vi "Register Dynamic Status Change Event.vi"() -> ()   [LabVIEW 2017]
doc: "------------- lvcsm -------------\n[CSMStates]\nItem 0 = \"Event Structure\"\nItem 1 = \"Idle\"\nItem 2 = \"CSM Documentation\"\nItem 3 = \"VI Reference\"\nItem 4 = \"Error Handler\"\nItem 5 = \"Critical Error\"\nItem 6 = \"Target Timeout Error\"\nItem 7 = \"Target Error\"\nItem 8 = \"Async Response\"\nItem 9 = \"Response\"\nItem 10 = \"Async Message Posted\"\nItem 11 = \"Initialize Core Data\"\nItem 12 = \"Exit\"\nItem 13 = \"Data: Initialize\"\nItem 14 = \"Data: Cleanup\"\nItem 15 = \"Events: Register\"\nItem 16 = \"Events: Unregister\"\nItem 17 = \"UI: Initialize\"\nItem 18 = \"UI: Cursor Set\"\nItem 19 = \"UI: Front Panel State\"\nItem 20 = \"Macro: Initialize\"\nItem 21 = \"Macro: Exit\"\nItem 22 = \"API: API1\"\nItem 23 = \"API: API2\"\nItem 24 = \"DoSth: DoA\"\nItem 25 = \"Update Status Changed\"\nItem 26 = \"DoSth: DoB\"\nItem 27 = \"Handler: Error Occurred\"\n\n[CSMStatus]"
uses:
  user.lib/_NEVSTOP/Communicable State Machine(CSM)/_Support/Common/Format Timestamp.vi
  user.lib/_NEVSTOP/Communicable State Machine(CSM)/_Polymophic/Build Synchronous Message with Arguments.vi
  user.lib/_NEVSTOP/Communicable State Machine(CSM)/Communicable State Machine.lvlib
  examples/NEVSTOP/Communicable State Machine(CSM)/1. Create a reuse Module/1. Create a reuse Module.lvlib
panel:
  in  "unRegister":bool
  in  "Register":bool
  out "State History 2":string
  in  "Start SubModule":bool
  out "State History":string
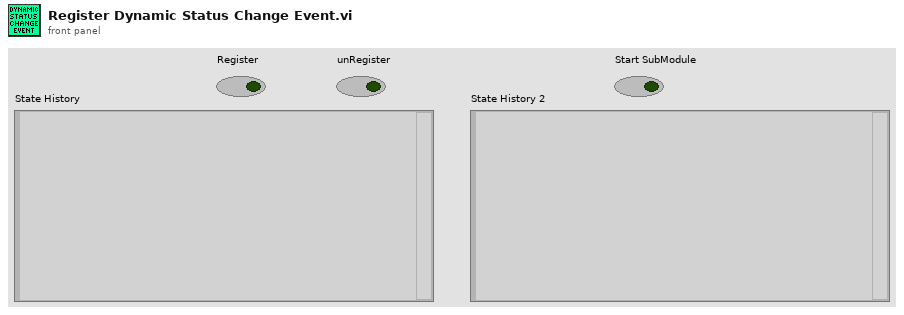
[diagram p1: front panel]
types:
  T1 = enum32{"Invalid", "Standard", "Closed", "Hidden", "Minimized", "Maximized"}
  T2 = enum32{"invalid app kind", "Development System", "Run Time System", "Student Edition", "Embedded LabVIEW", "Evaluation", "Custom"}
  T3 = typedef "Communicable State Machine.lvlib/_CSM_Response Source Message.ctl" = cluster{"‘State":string, "’Arguments":string, "’Error":errorcluster}
  T4 = cluster{"Current VI Reference":refnum<vi>, "Close Panel on Exit?":bool}
  T5 = cluster{"Core":cluster{"Current VI Reference":refnum<vi>, "Close Panel on Exit?":bool}, "Your Boolean data":bool, "Your string data":string}
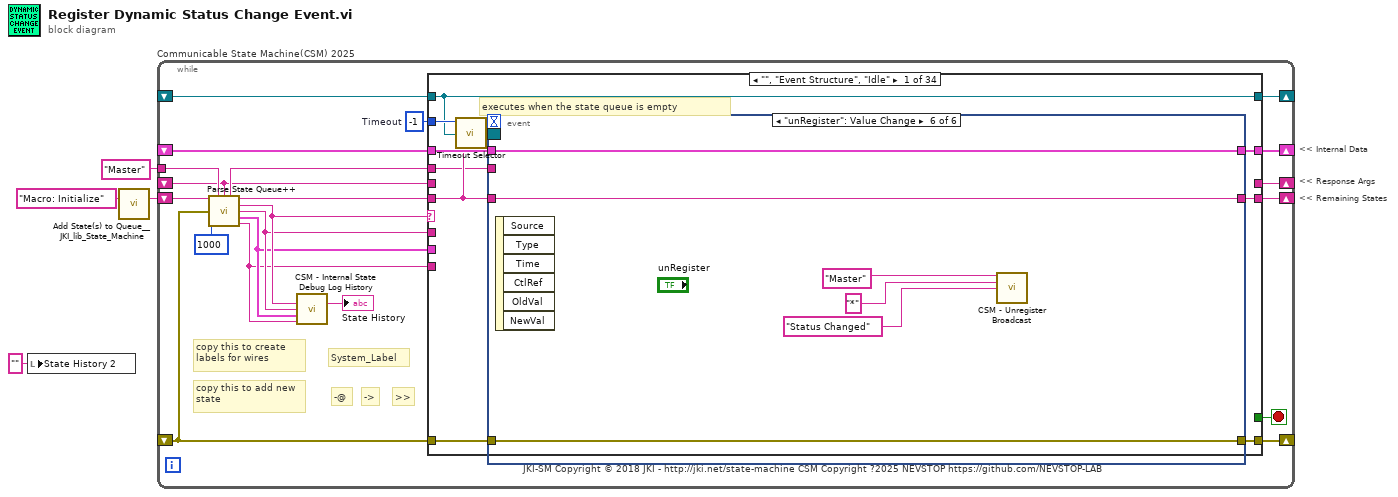
[diagram p0: block diagram]
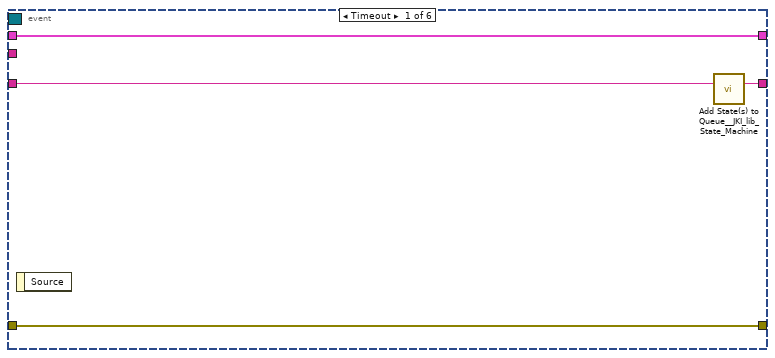
[diagram p2: hidden frame]
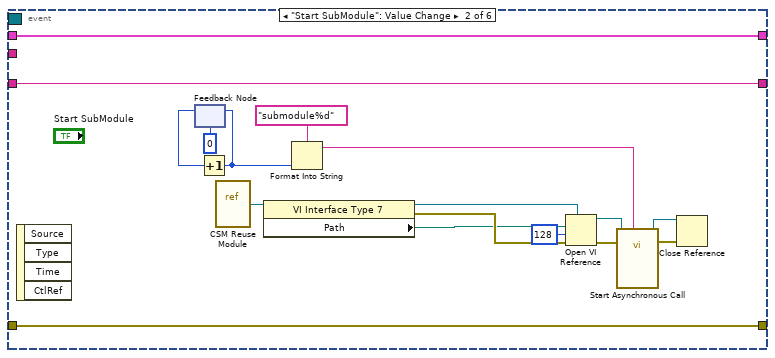
[diagram p3: hidden frame]
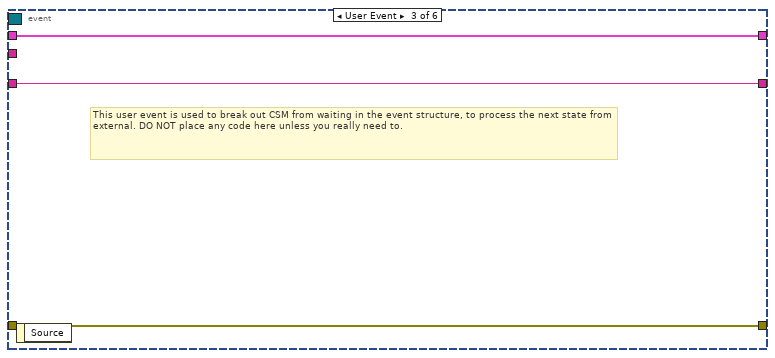
[diagram p4: hidden frame]
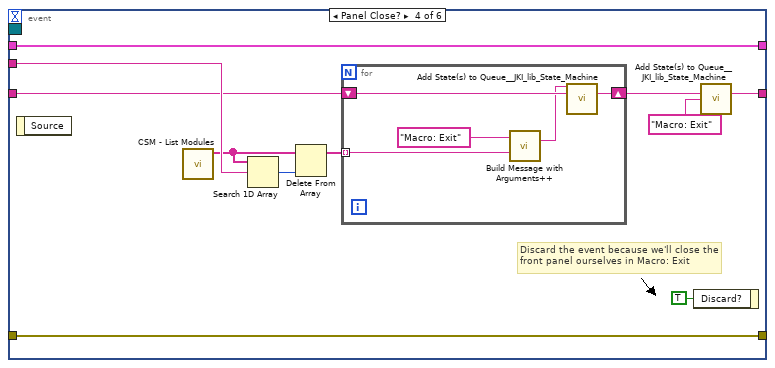
[diagram p5: hidden frame]
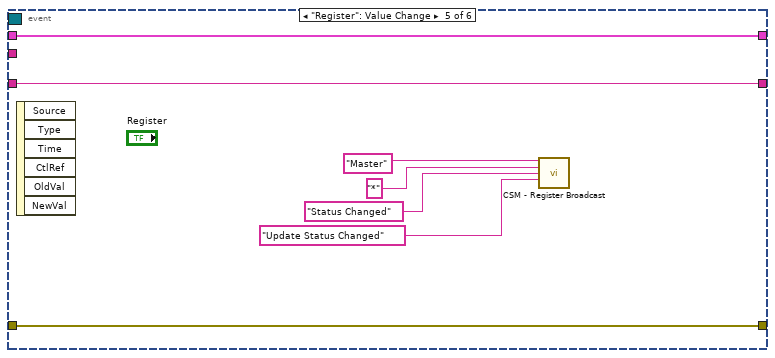
[diagram p6: hidden frame]
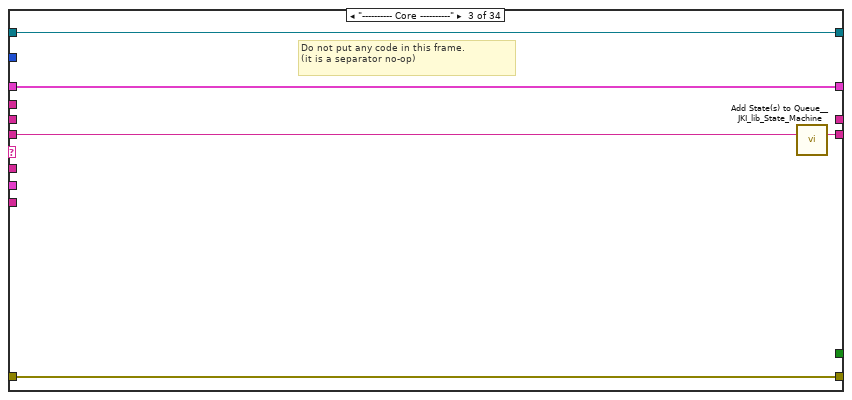
[diagram p8: hidden frame]
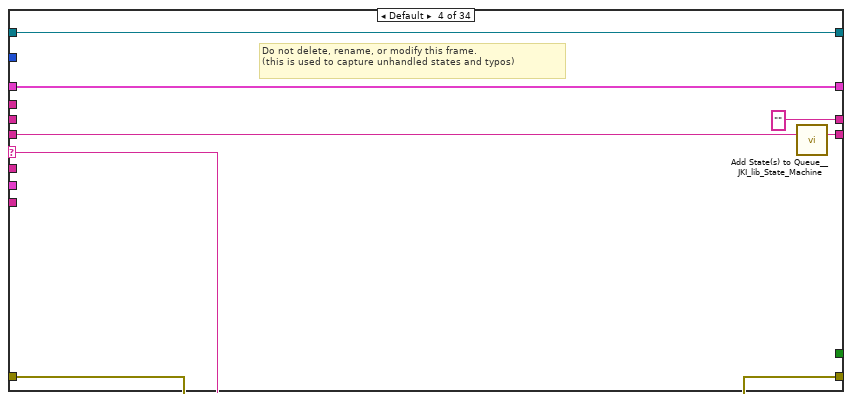
[diagram p9: hidden frame]
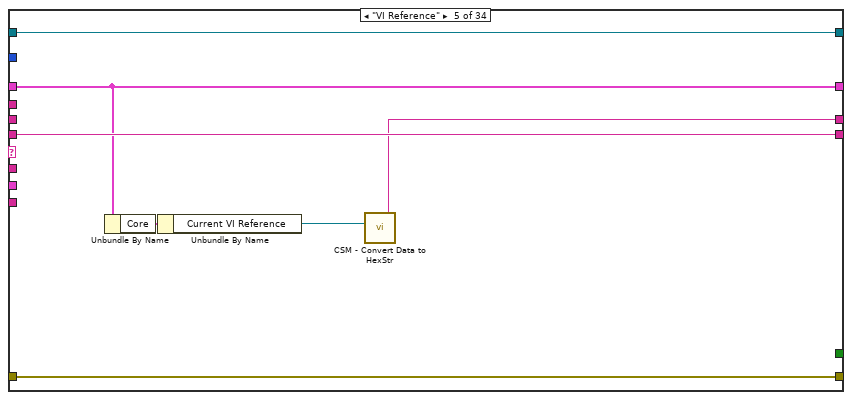
[diagram p10: hidden frame]
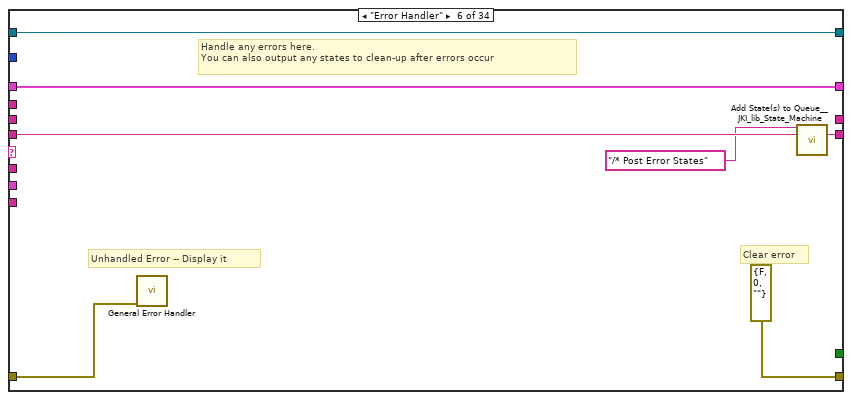
[diagram p11: hidden frame]
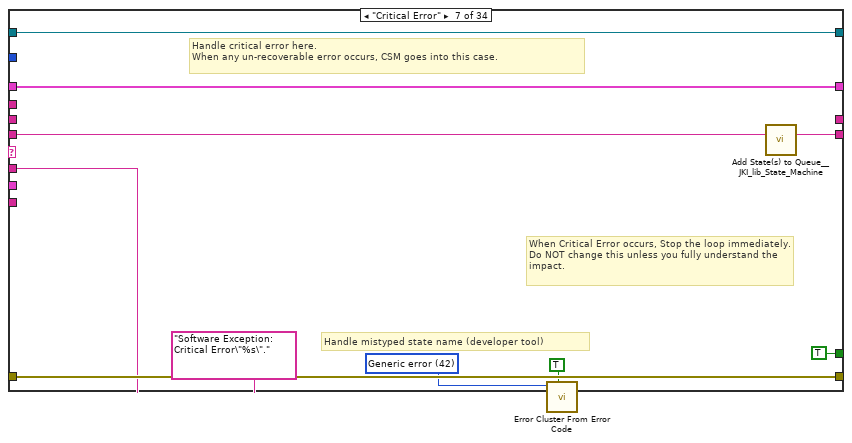
[diagram p12: hidden frame]
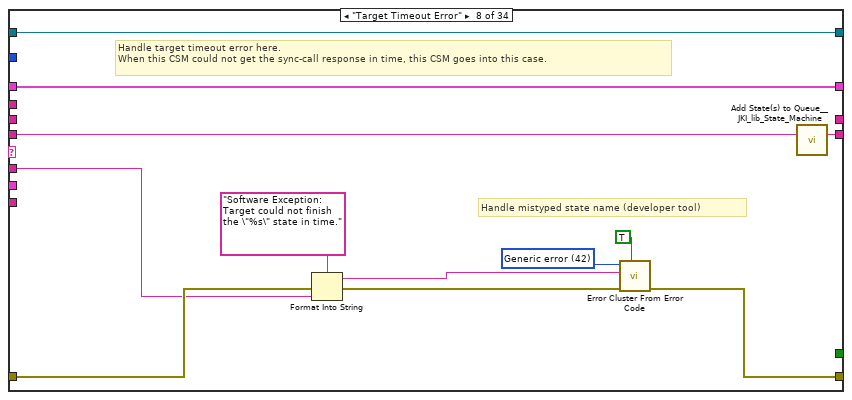
[diagram p13: hidden frame]
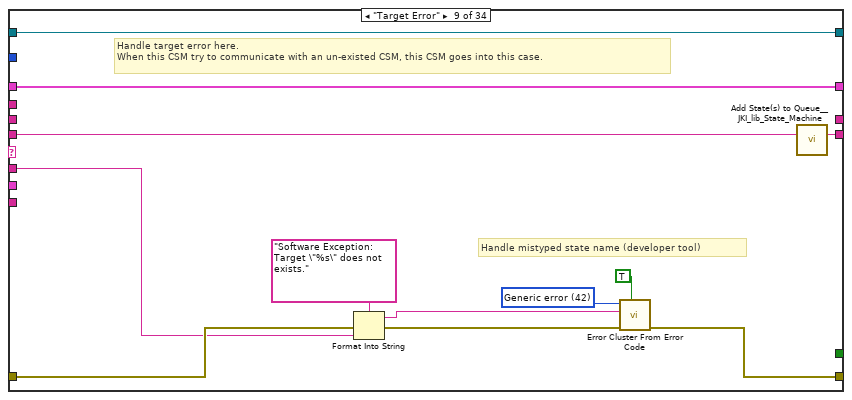
[diagram p14: hidden frame]
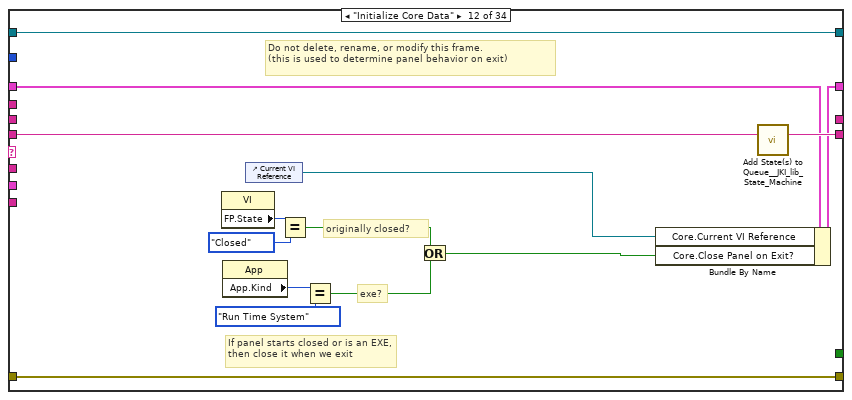
[diagram p17: hidden frame]
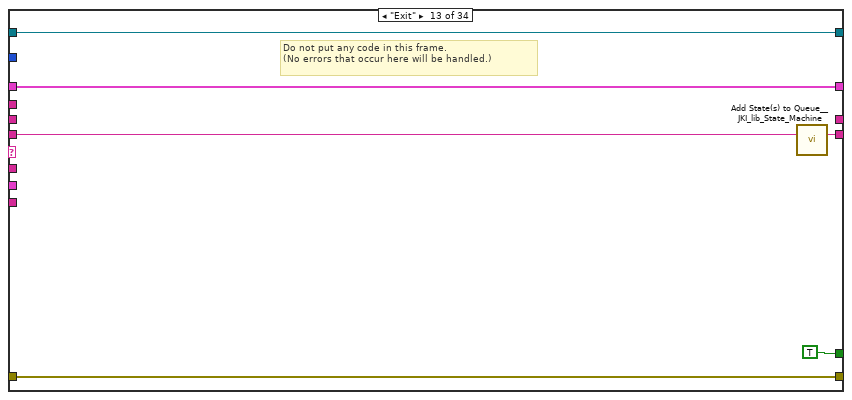
[diagram p18: hidden frame]
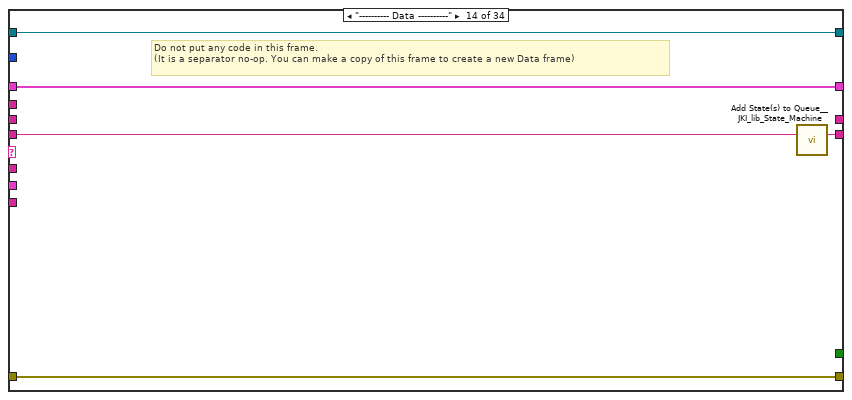
[diagram p19: hidden frame]
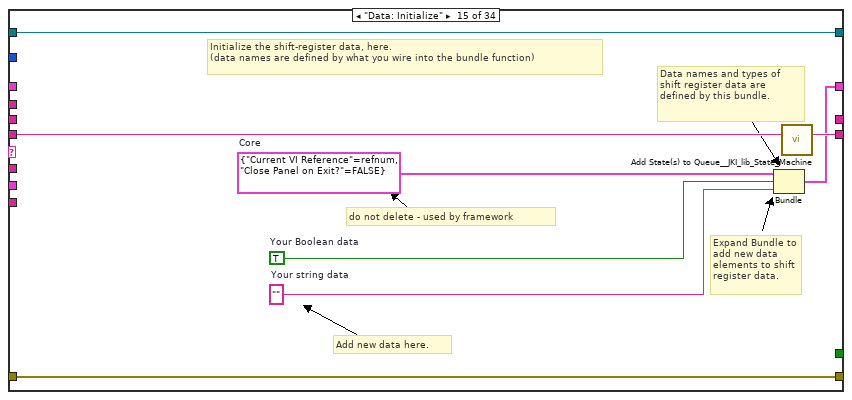
[diagram p20: hidden frame]
diagram:
  # "<< Internal Data"
  # "<< Response Args"
  # "<< Remaining States"
  n1 = local write "State History 2"("" ("State History 2")) -> ()
  n2 = call <vilib>:"Add State(s) to Queue__JKI_lib_State_Machine.vi"("State(s) in (\"\")"="Macro: Initialize") -> ("States Out"=w4:string)  [unwired: 14 in]
  n3 = while "Communicable State Machine(CSM) 2025" {
    shift-right: [w20] -> _
    shift-left: _ -> [w19]
    shift-right: [w23] -> _
    shift-left: _ -> [w17]
    shift-right: [w22] -> _
    shift-left: w4 -> [w24]
    tunnel: "Master" ("Name(\"\" to use uuid)") -> [w12]
    shift-right: [w15] -> _
    shift-left: _ -> [w6]
    shift-right: [w14] -> _
    shift-left: _ -> [w13]
    stop <- w21 stop-if-true
    w18 = -1  # Timeout
    # "JKI-SM Copyright © 2018 JKI - http://jki.net/state-machine CSM Copyright ?2025 NEVSTOP https://github.com/NEVSTOP-LAB"
    # "copy this to add new state"
    # ">>"
    # "->"
    # "-@"
    # "copy this to create labels for wires"
    # "System_Label"
    n4 = call "Parse State Queue++.vi"("State Queue"=w24, "Name (\"\" to Use UUID)"=w12, "Response Arguments"=w6, "Previous Error"=w17, "Response Timeout (-2 Use Global Settings)"=1000 ("Response Timeout(1000ms)")) -> ("Name Used"=w7:string, "Remaining States"=w25:string, "Current State"=w11:string, "Arguments"=w10:string, "Additional Information"=w9:T3, "Source CSM"=w8:string)  [unwired: 5 in]
    n5 = call "CSM - Internal State Debug Log History.vi"("State"=w11, "Arguments (\"\")"=w10, ">> Response Source Message >>"=w9, "Source (\"\")"=w8) -> ("Debug Log"=→"State History":string)  [unwired: 11 in]
    n6 = case shown="\"\", \"Event Structure\", \"Idle\"" w11 {
      selector: w11 -> [_ _ _ w100 _ _ _ _ _ _ _ _ _ _ _ _ _ _ _ _ _ _ _ _ _ _ _ _ _ _ _ _ _ _]
      tunnel: w25 -> [w27 w91 w97 w104 w116 w124 w134 w142 w154 w163 w167 w182 w188 w193 w201 w208 w213 w219 w223 w229 w234 w241 w253 w323 w329 w340 w343 w348 w354 w362 w368 w376 w383 w398]
      tunnel: w10 -> [_ _ _ _ _ _ w127 w138 w150 _ _ _ _ _ _ _ _ _ _ _ _ w236 w247 _ _ _ _ _ w351 _ _ w370 _ w395]
      tunnel: w19 -> [w34 w90 w94 w102 w115 w121 w135 w140 w152 w162 w166 w175 w186 w190 _ w203 w210 w218 w222 w226 w232 w239 w249 w320 w326 w337 w342 w347 w353 w359 w365 w375 w380 w397]
      tunnel: [w33 w92 w95 w106 w117 errorcluster {"status"=FALSE, "code"=0, "source"=""} ("error out") w136 w144 w156 w164 w168 w179 w185 w191 w198 w204 w211 w214 w221 w227 w231 w237 w250 w321 w327 w338 w344 w349 w355 w360 w366 w377 w381 w399] -> w23
      tunnel: w17 -> [w32 w92 w95 w105 w117 w120 w136 w143 w155 w164 w168 w179 w185 w191 w198 w205 w211 _ w224 w227 w231 w238 w251 w321 w327 w338 w344 w349 w355 w360 w366 w377 w381 w399]
      tunnel: [w35 w91 w96 w103 w116 w123 w133 w141 w153 w163 w167 w181 w187 w192 w200 w207 w212 w219 w223 w228 w233 w240 w252 w322 w328 w339 w343 w348 w354 w361 w367 w376 w382 w398] -> w22
      tunnel: [_ _ _ _ _ _ TRUE _ _ _ _ _ TRUE _ _ _ _ _ _ _ _ _ _ _ _ _ _ _ _ _ _ _ _ _] -> w21
      tunnel: [w31 w90 w94 w102 w115 w121 w135 w140 w152 w162 w166 w180 w186 w190 w199 w203 w210 w218 w222 w226 w232 w239 w249 w320 w326 w337 w342 w347 w353 w359 w365 w375 w380 w397] -> w20
      tunnel: w18 -> [w30 _ _ _ _ _ _ _ _ _ _ _ _ _ _ _ _ _ _ _ _ _ _ _ _ _ _ _ _ _ _ _ _ _]
      tunnel: w8 -> [_ _ _ _ _ _ _ _ _ _ _ _ _ _ _ _ _ _ _ _ _ _ _ _ _ _ _ _ _ _ _ w371 _ w390]
      tunnel: w9 -> [_ _ _ _ _ _ _ _ _ _ _ _ _ _ _ _ _ _ _ _ _ _ _ _ _ _ _ _ _ _ _ _ _ w389]
      tunnel: [_ _ _ "" w111 _ _ _ _ _ _ _ _ _ _ _ _ _ _ _ _ _ _ _ _ _ _ "API1 Response" w350 _ "DoA Finished" _ "DoB Finished" _] -> w15
      tunnel: [w29 w89 w93 w98 w114 w118 w125 w137 w149 w161 w165 w169 w183 w189 w194 w202 w209 w217 w220 w225 w230 w235 w246 w319 w324 w330 w341 w346 w352 w358 w364 w374 w379 w396] -> w14
      tunnel: w13 -> [w29 w89 w93 w98 w114 w118 w125 w137 w149 w161 w165 w169 w183 w189 w194 w202 w209 _ w220 w225 w230 w235 w246 w319 w324 w330 w341 w346 w352 w358 w364 w374 w379 w396]
      tunnel: w7 -> [w26 _ _ _ _ _ _ _ _ _ _ _ _ _ _ _ _ w216 _ _ _ _ _ _ _ _ _ _ _ _ _ _ _ _]
      tunnel: w6 -> [_ _ _ _ _ _ _ _ _ _ _ _ _ _ _ _ _ _ _ _ _ _ _ _ _ _ _ _ _ _ _ _ _ _]
      frame "", "Event Structure", "Idle" {
        # "executes when the state queue is empty"
        n7 = call "Timeout Selector.vi"("Remaining States"=w27, "Timeout Expected"=w30) -> ("Timeout"=w28:i32)  [unwired: 5 in]
        n8 = event shown="[5] \"unRegister\": Value Change" {
          selector: w29 -> [_ _ _ _ _ _]
          dyn-events: _ -> [_ _ _ _ _ _]
          timeout: w28 -> [_ _ _ _ _ _]
          tunnel: w27 -> [w39 w56 w58 w61 w82 w88]
          tunnel: [w38 w56 w58 w70 w82 w88] -> w35
          tunnel: w34 -> [w36 w54 w59 w68 w80 w86]
          tunnel: [w37 w55 w57 w69 w81 w87] -> w33
          tunnel: w32 -> [w37 w55 w57 w69 w81 w87]
          tunnel: [w36 w54 w59 w68 w80 w86] -> w31
          tunnel: w26 -> [_ _ _ w66 _ _]
          event Timeout {
            n9 = event-data() -> ()  [unwired: 1 in, 1 out]
            n10 = call <vilib>:"Add State(s) to Queue__JKI_lib_State_Machine.vi"("State(s) in (\"\")"=w39) -> ("States Out"=w38:string)  [unwired: 14 in]
          }
          event "Start SubModule": Value Change {
            n11 = event-data() -> ()  [unwired: 1 in, 4 out]
            n12 = feedback #1(0 ("Response Timeout(1000ms)")) -> (w52:i32)
            n13 = Increment(x=w52) -> (x+1=w42:i32)
            n14 = feedback-in #1(w42) -> ()
            n15 = vi-ref "CSM Reuse Module.vi"() -> (w44:refnum<vi>)
            n16 = property class="VI Interface Type 7"(reference=w44) -> (reference out=w48:refnum<vi>, error out=w46:errorcluster, "Path"=w45:path)  [unwired: 1 in]
            n17 = Format Into String(format string="submodule%d", w42) -> (resulting string=w40:string)  [unwired: 2 in, 1 out]
            n18 = Open VI Reference(type specifier VI Refnum (for type only)=w48, vi path=w45, options=128, error in (no error)=w46) -> (vi reference=w47:refnum<vi>, error out=w43:errorcluster)  [unwired: 2 in]
            n19 = call-by-ref "Start Asynchronous Call"(reference=w47, error in=w43, "Name(\"\" to use uuid)"=w40) -> (reference out=w50:refnum<vi>, error out=w49:errorcluster)  [unwired: 11 in]
            n20 = Close Reference(reference=w50, error in (no error)=w49) -> ()  [unwired: 1 out]
          }
          event User Event {
            # "This user event is used to break out CSM from waiting in the event structure, to process the next state from external. DO NOT place any code here unless you really need to."
            n21 = event-data() -> ()  [unwired: 1 in, 1 out]
          }
          event Panel Close? {
            # "Discard the event because we'll close the front panel ourselves in Macro: Exit"
            n22 = event-data() -> ()  [unwired: 1 in, 1 out]
            n23 = call "CSM - List Modules.vi"() -> ("Module Names"=w65:string[])  [unwired: 10 in, 1 out]
            n24 = Search 1D Array(1D array=w65, element=w66) -> (index of element=w64:i32)  [unwired: 1 in]
            n25 = Delete From Array(array=w65, index=w64) -> (array with subset deleted=w63:string[])  [unwired: 1 in, 1 out]
            n26 = for {
              tunnel: w63 -> [w75] mode=indexing
              shift-right: [w73] -> w62
              shift-left: w61 -> [w72]
              n27 = call-poly "Build Message with Arguments++.vi"("State With Arguments"="Macro: Exit", "Target Module (\"\")"=w75) -> ("CSM Message String"=w71:string)  [unwired: 13 in]
              n28 = call <vilib>:"Add State(s) to Queue__JKI_lib_State_Machine.vi"("State(s) in Front (\"\")"=w71, "State(s) in (\"\")"=w72) -> ("States Out"=w73:string)  [unwired: 13 in]
            }
            n29 = event-data("Discard?"=TRUE) -> ()  [unwired: 1 in, 1 out]
            n30 = call <vilib>:"Add State(s) to Queue__JKI_lib_State_Machine.vi"("State(s) in (\"\")"=w62, "State(s) at Back (\"\")"="Macro: Exit") -> ("States Out"=w70:string)  [unwired: 13 in]
          }
          event "Register": Value Change {
            n31 = event-data() -> ()  [unwired: 1 in, 6 out]
            n32 = call "CSM - Register Broadcast.vi"("CSM Name(Empty for Broadcast Event)"="Master" ("Source CSM Name"), "Source CSM Name (* as Default)"="*" ("Name(\"\" to use uuid)"), "Trigger"="Status Changed" ("Message"), "API (If \"\", Same as Trigger)"="Update Status Changed" ("Response Message (if \"\", same as Source Message)")) -> ()  [unwired: 10 in, 2 out]
          }
          event "unRegister": Value Change {
            n33 = event-data() -> ()  [unwired: 1 in, 6 out]
            n34 = call "CSM - Unregister Broadcast.vi"("CSM Name(Empty for Broadcast Event)"="Master" ("Source CSM Name"), "Source CSM Name (* as Default)"="*" ("Name(\"\" to use uuid)"), "Trigger"="Status Changed" ("Message")) -> ()  [unwired: 11 in, 2 out]
          }
        }
      }
      frame "CSM Documentation" {
        # "CSM Documentation"
      }
      frame "---------- Core ----------" {
        # "Do not put any code in this frame.\n(it is a separator no-op)"
        n35 = call <vilib>:"Add State(s) to Queue__JKI_lib_State_Machine.vi"("State(s) in (\"\")"=w97) -> ("States Out"=w96:string)  [unwired: 14 in]
      }
      frame Default {
        w109 = 42 items=["No error", "Argument error", "Memory is full", "Out of zone", "End of file", "File already open", "Generic file I/O error", "File not found", "File permission error", "Disk is full", "Duplicate path", "Too many files open", "System feature not enabled", "Resource file not found", "Cannot add resource", "Resource not found", "Image not found", "Image memory error", "Pen does not exist", "Config type invalid", "Config token not found", "Config parse error", "Config memory error", "Bad external code format", "Bad external code offset", "External code not present", "Null window", "Destroy window error", "Null menu", "Print aborted", "Bad print record", "Print driver error", "Windows error during printing", "Memory error during printing", "Print dialog error", "Generic print error", "Invalid device refnum", "Device not found", "Device parameter error", "Device unit error", "Cannot open device", "Device call aborted", "Generic error", "Cancelled by user", "Object ID too low", "Object ID too high", "Object not in heap", "Unknown heap", "Unknown object (invalid DefProc)", "Unknown object (DefProc not in table)", "Message out of range", "Invalid (null) method", "Unknown message", "Manager call not supported", "Bad address", "Network operation in progress", "Network operation timed out", "Connection is busy", "Network attribute not supported", "Network error", "Address in use", "System out of memory", "Connection aborted", "Connection refused", "Not connected", "Already connected", "Connection closed", "Initialization error (interapplication manager)", "Bad occurrence", "Wait on unbound occurrence handler", "Occurrence queue overflow", "Datalog type conflict", "Unused", "Unrecognized type (interapplication manager)", "Memory corrupt", "Failed to make temporary DLL", "Old CIN version", "Drag socket not found", "Failed to load drop-object", "Failed to register OLE object", "Failed to release OLE object", "Format specifier type mismatch", "Unknown format specifier", "Too few format specifiers", "Too many format specifiers", "Scan failed", "Newer CIN version", "Error converting to variant", "Runtime menu error", "Password tampered", "Variant attribute not found", "Incompatible variant data type", "Event data is not available", "Event Store is not present", "Occurrence is not found", "Event Queue is not created", "Event info is not available", "Refnum passed is NULL", "Error retrieving Class GUID", "Error retrieving CoClass GUID", "Error retrieving TypeLib GUID.", "Bad built application magic bytes.", "Specific driver is different from the specific driver associated with the Logical Name.", "There is no session opened to the class driver.", "Max Error", "MAX - Error with config objects", "MAX - Error loading configuration", "MAX - Group not supported"]
        # "Do not delete, rename, or modify this frame.\n(this is used to capture unhandled states and typos)"
        # "Handle mistyped state name (developer tool)"
        n36 = Format Into String(format string="Software Exception: Unhandled State \"%s\"." ("message"), error in=w105, w100) -> (resulting string=w108:string, error out=w107:errorcluster)  [unwired: 1 in]
        n37 = call <vilib>:"Error Cluster From Error Code.vi"("show call chain? (False)"=TRUE, "error in (no error)"=w107, "error message (\"\")"=w108, "error code (0)"=w109) -> ("error out"=w106:errorcluster)  [unwired: 5 in]
        n38 = call <vilib>:"Add State(s) to Queue__JKI_lib_State_Machine.vi"("State(s) in (\"\")"=w104) -> ("States Out"=w103:string)  [unwired: 14 in]
      }
      frame "VI Reference" {
        n39 = Unbundle By Name(w115) -> ("Core"=w113:T4)
        n40 = Unbundle By Name(w113) -> ("Current VI Reference"=w112:refnum<vi>)
        n41 = call "CSM - Convert Data to HexStr.vi"("Variant"=w112) -> ("HEX String (0-9,A-F)"=w111:string)  [unwired: 8 in]
      }
      frame "Error Handler" {
        # "Unhandled Error -- Display it"
        # "Handle any errors here.\nYou can also output any states to clean-up after errors occur"
        # "Clear error"
        n42 = call <vilib>:"General Error Handler.vi"("error in (no error)"=w120) -> ()  [unwired: 10 in, 5 out]
        n43 = call <vilib>:"Add State(s) to Queue__JKI_lib_State_Machine.vi"("State(s) in Front (\"\")"="/* Post Error States", "State(s) in (\"\")"=w124) -> ("States Out"=w123:string)  [unwired: 13 in]
      }
      frame "Critical Error" {
        w131 = 42 items=["No error", "Argument error", "Memory is full", "Out of zone", "End of file", "File already open", "Generic file I/O error", "File not found", "File permission error", "Disk is full", "Duplicate path", "Too many files open", "System feature not enabled", "Resource file not found", "Cannot add resource", "Resource not found", "Image not found", "Image memory error", "Pen does not exist", "Config type invalid", "Config token not found", "Config parse error", "Config memory error", "Bad external code format", "Bad external code offset", "External code not present", "Null window", "Destroy window error", "Null menu", "Print aborted", "Bad print record", "Print driver error", "Windows error during printing", "Memory error during printing", "Print dialog error", "Generic print error", "Invalid device refnum", "Device not found", "Device parameter error", "Device unit error", "Cannot open device", "Device call aborted", "Generic error", "Cancelled by user", "Object ID too low", "Object ID too high", "Object not in heap", "Unknown heap", "Unknown object (invalid DefProc)", "Unknown object (DefProc not in table)", "Message out of range", "Invalid (null) method", "Unknown message", "Manager call not supported", "Bad address", "Network operation in progress", "Network operation timed out", "Connection is busy", "Network attribute not supported", "Network error", "Address in use", "System out of memory", "Connection aborted", "Connection refused", "Not connected", "Already connected", "Connection closed", "Initialization error (interapplication manager)", "Bad occurrence", "Wait on unbound occurrence handler", "Occurrence queue overflow", "Datalog type conflict", "Unused", "Unrecognized type (interapplication manager)", "Memory corrupt", "Failed to make temporary DLL", "Old CIN version", "Drag socket not found", "Failed to load drop-object", "Failed to register OLE object", "Failed to release OLE object", "Format specifier type mismatch", "Unknown format specifier", "Too few format specifiers", "Too many format specifiers", "Scan failed", "Newer CIN version", "Error converting to variant", "Runtime menu error", "Password tampered", "Variant attribute not found", "Incompatible variant data type", "Event data is not available", "Event Store is not present", "Occurrence is not found", "Event Queue is not created", "Event info is not available", "Refnum passed is NULL", "Error retrieving Class GUID", "Error retrieving CoClass GUID", "Error retrieving TypeLib GUID.", "Bad built application magic bytes.", "Specific driver is different from the specific driver associated with the Logical Name.", "There is no session opened to the class driver.", "Max Error", "MAX - Error with config objects", "MAX - Error loading configuration", "MAX - Group not supported"]
        # "Handle critical error here.\nWhen any un-recoverable error occurs, CSM goes into this case."
        # "When Critical Error occurs, Stop the loop immediately. Do NOT change this unless you fully understand the impact."
        # "Handle mistyped state name (developer tool)"
        n44 = Format Into String(format string="Software Exception: Critical Error\"%s\"." ("message"), w127) -> (resulting string=w130:string, error out=w129:errorcluster)  [unwired: 2 in]
        n45 = call <vilib>:"Error Cluster From Error Code.vi"("show call chain? (False)"=TRUE, "error in (no error)"=w129, "error message (\"\")"=w130, "error code (0)"=w131) -> ()  [unwired: 5 in, 1 out]
        n46 = call <vilib>:"Add State(s) to Queue__JKI_lib_State_Machine.vi"("State(s) in (\"\")"=w134) -> ("States Out"=w133:string)  [unwired: 14 in]
      }
      frame "Target Timeout Error" {
        w147 = 42 items=["No error", "Argument error", "Memory is full", "Out of zone", "End of file", "File already open", "Generic file I/O error", "File not found", "File permission error", "Disk is full", "Duplicate path", "Too many files open", "System feature not enabled", "Resource file not found", "Cannot add resource", "Resource not found", "Image not found", "Image memory error", "Pen does not exist", "Config type invalid", "Config token not found", "Config parse error", "Config memory error", "Bad external code format", "Bad external code offset", "External code not present", "Null window", "Destroy window error", "Null menu", "Print aborted", "Bad print record", "Print driver error", "Windows error during printing", "Memory error during printing", "Print dialog error", "Generic print error", "Invalid device refnum", "Device not found", "Device parameter error", "Device unit error", "Cannot open device", "Device call aborted", "Generic error", "Cancelled by user", "Object ID too low", "Object ID too high", "Object not in heap", "Unknown heap", "Unknown object (invalid DefProc)", "Unknown object (DefProc not in table)", "Message out of range", "Invalid (null) method", "Unknown message", "Manager call not supported", "Bad address", "Network operation in progress", "Network operation timed out", "Connection is busy", "Network attribute not supported", "Network error", "Address in use", "System out of memory", "Connection aborted", "Connection refused", "Not connected", "Already connected", "Connection closed", "Initialization error (interapplication manager)", "Bad occurrence", "Wait on unbound occurrence handler", "Occurrence queue overflow", "Datalog type conflict", "Unused", "Unrecognized type (interapplication manager)", "Memory corrupt", "Failed to make temporary DLL", "Old CIN version", "Drag socket not found", "Failed to load drop-object", "Failed to register OLE object", "Failed to release OLE object", "Format specifier type mismatch", "Unknown format specifier", "Too few format specifiers", "Too many format specifiers", "Scan failed", "Newer CIN version", "Error converting to variant", "Runtime menu error", "Password tampered", "Variant attribute not found", "Incompatible variant data type", "Event data is not available", "Event Store is not present", "Occurrence is not found", "Event Queue is not created", "Event info is not available", "Refnum passed is NULL", "Error retrieving Class GUID", "Error retrieving CoClass GUID", "Error retrieving TypeLib GUID.", "Bad built application magic bytes.", "Specific driver is different from the specific driver associated with the Logical Name.", "There is no session opened to the class driver.", "Max Error", "MAX - Error with config objects", "MAX - Error loading configuration", "MAX - Group not supported"]
        # "Handle target timeout error here.\nWhen this CSM could not get the sync-call response in time, this CSM goes into this case."
        # "Handle mistyped state name (developer tool)"
        n47 = Format Into String(format string="Software Exception: Target could not finish the \"%s\" state in time." ("message"), error in=w143, w138) -> (resulting string=w146:string, error out=w145:errorcluster)  [unwired: 1 in]
        n48 = call <vilib>:"Error Cluster From Error Code.vi"("show call chain? (False)"=TRUE, "error in (no error)"=w145, "error message (\"\")"=w146, "error code (0)"=w147) -> ("error out"=w144:errorcluster)  [unwired: 5 in]
        n49 = call <vilib>:"Add State(s) to Queue__JKI_lib_State_Machine.vi"("State(s) in (\"\")"=w142) -> ("States Out"=w141:string)  [unwired: 14 in]
      }
      frame "Target Error" {
        w159 = 42 items=["No error", "Argument error", "Memory is full", "Out of zone", "End of file", "File already open", "Generic file I/O error", "File not found", "File permission error", "Disk is full", "Duplicate path", "Too many files open", "System feature not enabled", "Resource file not found", "Cannot add resource", "Resource not found", "Image not found", "Image memory error", "Pen does not exist", "Config type invalid", "Config token not found", "Config parse error", "Config memory error", "Bad external code format", "Bad external code offset", "External code not present", "Null window", "Destroy window error", "Null menu", "Print aborted", "Bad print record", "Print driver error", "Windows error during printing", "Memory error during printing", "Print dialog error", "Generic print error", "Invalid device refnum", "Device not found", "Device parameter error", "Device unit error", "Cannot open device", "Device call aborted", "Generic error", "Cancelled by user", "Object ID too low", "Object ID too high", "Object not in heap", "Unknown heap", "Unknown object (invalid DefProc)", "Unknown object (DefProc not in table)", "Message out of range", "Invalid (null) method", "Unknown message", "Manager call not supported", "Bad address", "Network operation in progress", "Network operation timed out", "Connection is busy", "Network attribute not supported", "Network error", "Address in use", "System out of memory", "Connection aborted", "Connection refused", "Not connected", "Already connected", "Connection closed", "Initialization error (interapplication manager)", "Bad occurrence", "Wait on unbound occurrence handler", "Occurrence queue overflow", "Datalog type conflict", "Unused", "Unrecognized type (interapplication manager)", "Memory corrupt", "Failed to make temporary DLL", "Old CIN version", "Drag socket not found", "Failed to load drop-object", "Failed to register OLE object", "Failed to release OLE object", "Format specifier type mismatch", "Unknown format specifier", "Too few format specifiers", "Too many format specifiers", "Scan failed", "Newer CIN version", "Error converting to variant", "Runtime menu error", "Password tampered", "Variant attribute not found", "Incompatible variant data type", "Event data is not available", "Event Store is not present", "Occurrence is not found", "Event Queue is not created", "Event info is not available", "Refnum passed is NULL", "Error retrieving Class GUID", "Error retrieving CoClass GUID", "Error retrieving TypeLib GUID.", "Bad built application magic bytes.", "Specific driver is different from the specific driver associated with the Logical Name.", "There is no session opened to the class driver.", "Max Error", "MAX - Error with config objects", "MAX - Error loading configuration", "MAX - Group not supported"]
        # "Handle target error here.\nWhen this CSM try to communicate with an un-existed CSM, this CSM goes into this case."
        # "Handle mistyped state name (developer tool)"
        n50 = Format Into String(format string="Software Exception: Target \"%s\" does not exists." ("message"), error in=w155, w150) -> (resulting string=w158:string, error out=w157:errorcluster)  [unwired: 1 in]
        n51 = call <vilib>:"Error Cluster From Error Code.vi"("show call chain? (False)"=TRUE, "error in (no error)"=w157, "error message (\"\")"=w158, "error code (0)"=w159) -> ("error out"=w156:errorcluster)  [unwired: 5 in]
        n52 = call <vilib>:"Add State(s) to Queue__JKI_lib_State_Machine.vi"("State(s) in (\"\")"=w154) -> ("States Out"=w153:string)  [unwired: 14 in]
      }
      frame "Async Response", "Response" {
        # "Handle Async-call Response (\"Async Response\" for ->)"
        # "Handle Sync-call Response (\"Response\" for @)"
        # "After Message is executed, CSM goes to this state for receive the response. \n    For Async Message(->), \"Async Response\" is used. This CSM will goes to \"Async Message Posted\" immediately and receive the \"Async Response\" after the callee finishes the message.\n    For Sync Message(@),  This CSM will wait until the message is done and immediately goes to \"Response\""
      }
      frame "Async Message Posted" {
        # "Handle post action for async message (->)."
        # "After Async Message is posted (->), CSM goes to this state for post-action. You can use Argument - State to tell which Async Message is called."
      }
      frame "Initialize Core Data" {
        # "Do not delete, rename, or modify this frame.\n(this is used to determine panel behavior on exit)"
        # "originally closed?"
        # "exe?"
        # "If panel starts closed or is an EXE, then close it when we exit"
        n53 = property class="VI"() -> ("FP.State"=w172:T1)  [unwired: 2 in, 2 out]
        n54 = property class="App"() -> ("App.Kind"=w178:T2)  [unwired: 2 in, 2 out]
        n55 = control-ref of="Current VI Reference"() -> (w173:refnum<vi>)
        n56 = Equal?(x=w172, y=T1."Closed" ("Front Panel Window:State")) -> (x = y?=w170:bool)
        n57 = Equal?(x=w178, y=T2."Run Time System" ("Application:Kind")) -> (x = y?=w176:bool)
        n58 = Or(x=w170, y=w176) -> (x .or. y?=w174:bool)
        n59 = Bundle By Name(cluster=w175, "Core.Current VI Reference"=w173, "Core.Close Panel on Exit?"=w174) -> (w180:T5)
        n60 = call <vilib>:"Add State(s) to Queue__JKI_lib_State_Machine.vi"("State(s) in (\"\")"=w182) -> ("States Out"=w181:string)  [unwired: 14 in]
      }
      frame "Exit" {
        # "Do not put any code in this frame.\n(No errors that occur here will be handled.)"
        n61 = call <vilib>:"Add State(s) to Queue__JKI_lib_State_Machine.vi"("State(s) in (\"\")"=w188) -> ("States Out"=w187:string)  [unwired: 14 in]
      }
      frame "---------- Data ----------" {
        # "Do not put any code in this frame.\n(It is a separator no-op. You can make a copy of this frame to create a new Data frame)"
        n62 = call <vilib>:"Add State(s) to Queue__JKI_lib_State_Machine.vi"("State(s) in (\"\")"=w193) -> ("States Out"=w192:string)  [unwired: 14 in]
      }
      frame "Data: Initialize" {
        w195 = T4 {"Current VI Reference"=refnum, "Close Panel on Exit?"=FALSE}  # Core
        w197 = TRUE  # Your Boolean data
        w196 = ""  # Your string data
        # "do not delete - used by framework"
        # "Expand Bundle to add new data elements to shift register data."
        # "Add new data here."
        # "Data names and types of shift register data are defined by this bundle."
        # "Initialize the shift-register data, here.\n(data names are defined by what you wire into the bundle function)"
        n63 = Bundle("Core"=w195, "Your Boolean data"=w197, "Your string data"=w196) -> (w199:T5)  [unwired: 1 in]
        n64 = call <vilib>:"Add State(s) to Queue__JKI_lib_State_Machine.vi"("State(s) in (\"\")"=w201) -> ("States Out"=w200:string)  [unwired: 14 in]
      }
      frame "Data: Cleanup" {
        # "Cleanup any data and references, here.\n(this is called automatically, by the Macro: Exit)"
        n65 = Unbundle By Name(w203) -> ("Core.Current VI Reference"=w206:refnum<vi>)
        n66 = Close Reference(reference=w206, error in (no error)=w205) -> (error out=w204:errorcluster)
        n67 = call <vilib>:"Add State(s) to Queue__JKI_lib_State_Machine.vi"("State(s) in (\"\")"=w208) -> ("States Out"=w207:string)  [unwired: 14 in]
      }
      frame "---------- Events ----------" {
        # "Do not put any code in this frame.\n(It is a separator no-op. You can make a copy of this frame to create a new UI frame)"
        n68 = call <vilib>:"Add State(s) to Queue__JKI_lib_State_Machine.vi"("State(s) in (\"\")"=w213) -> ("States Out"=w212:string)  [unwired: 14 in]
      }
      frame "Events: Register" {
        # "Register message event to break Waiting in Event structure."
        n69 = call "CSM - Get New State Notifier Event.vi"("Name (\"\" to Use UUID)"=w216) -> ("error out"=w214:errorcluster, "New State Notifier Event"=w215:refnum<user-event>)  [unwired: 9 in]
        n70 = register-events(w215) -> (reference out=w217:refnum<event-registration>)  [unwired: 2 in, 1 out]
      }
      frame "Events: Unregister" {
        n71 = Unregister For Events(event registration refnum=w220, error in=w224) -> (error out=w221:errorcluster)
      }
      frame "---------- UI ----------" {
        # "Do not put any code in this frame.\n(It is a separator no-op. You can make a copy of this frame to create a new UI frame)"
        n72 = call <vilib>:"Add State(s) to Queue__JKI_lib_State_Machine.vi"("State(s) in (\"\")"=w229) -> ("States Out"=w228:string)  [unwired: 14 in]
      }
      frame "UI: Initialize" {
        # "Initialize the User Interface, here.\n(this is called automatically, by the Macro: Init)"
        n73 = call <vilib>:"Add State(s) to Queue__JKI_lib_State_Machine.vi"("State(s) in (\"\")"=w234) -> ("States Out"=w233:string)  [unwired: 14 in]
      }
      frame "UI: Cursor Set" {
        # "Argument"
        # "Set and Unset Cursor Busy.\n(Usage: \"UI: Cursor Set >> Busy|Idle\")"
        n74 = case shown="\"Idle\", Default" w236 {
          tunnel: w238 -> [w243 w245]
          tunnel: [w242 w244] -> w237
          frame "Idle", Default {
            n75 = call <vilib>:"Unset Busy.vi"("error in (no error)"=w243) -> ("error out"=w242:errorcluster)  [unwired: 10 in]
          }
          frame "Busy" {
            n76 = call <vilib>:"Set Busy.vi"("error in (no error)"=w245) -> ("error out"=w244:errorcluster)  [unwired: 9 in, 1 out]
          }
        }
        n77 = call <vilib>:"Add State(s) to Queue__JKI_lib_State_Machine.vi"("State(s) in (\"\")"=w241) -> ("States Out"=w240:string)  [unwired: 14 in]
      }
      frame "UI: Front Panel State" {
        # "Argument"
        # "Set Front Panel Open or Closed\n(Usage: \"UI: Front Panel State >> Open|Close\")"
        n78 = Unbundle By Name(w249) -> ("Core.Current VI Reference"=w248:refnum<vi>)
        n79 = case shown="\"Minimize\", \"Minimized\"" w247 {
          tunnel: w251 -> [w259 w274 w285 w298 w311]
          tunnel: [w261 w275 w287 w300 w313] -> w250
          tunnel: w248 -> [w260 w272 w286 w299 w312]
          frame "Open", "Standard", Default {
            w254 = T1."Standard" ("State")
            n80 = property class="VI"(reference=w260, error in=w259) -> (reference out=w257:refnum<vi>, error out=w258:errorcluster, "FP.State"=w256:T1)
            n81 = Not Equal?(x=w256, y=w254) -> (x != y?=w255:bool)
            n82 = case shown="True" w255 {
              tunnel: [w265 w267] -> w261
              tunnel: w258 -> [w264 w267]
              tunnel: w257 -> [w263 _]
              tunnel: w254 -> [w262 _]
              frame True {
                n83 = invoke class="VI" method="FP.Open"(reference=w263, error in=w264, "Activate"=TRUE, "State"=w262) -> (error out=w265:errorcluster)  [unwired: 1 in, 4 out]
              }
              frame False {
              }
            }
          }
          frame "Close", "Closed" {
            n84 = property class="VI"(reference=w272, error in=w274) -> (reference out=w271:refnum<vi>, error out=w273:errorcluster, "FP.State"=w269:T1)
            n85 = Not Equal?(x=w269, y=T1."Closed" ("Front Panel Window:State")) -> (x != y?=w268:bool)
            n86 = case shown="True" w268 {
              tunnel: [w276 w279] -> w275
              tunnel: w273 -> [w276 w278]
              tunnel: w271 -> [_ w277]
              frame False {
              }
              frame True {
                n87 = invoke class="VI" method="FP.Close"(reference=w277, error in=w278) -> (error out=w279:errorcluster)  [unwired: 1 in, 2 out]
              }
            }
          }
          frame "Hidden", "Hide" {
            w280 = T1."Hidden" ("State")
            n88 = property class="VI"(reference=w286, error in=w285) -> (reference out=w283:refnum<vi>, error out=w284:errorcluster, "FP.State"=w282:T1)
            n89 = Not Equal?(x=w282, y=w280) -> (x != y?=w281:bool)
            n90 = case shown="True" w281 {
              tunnel: [w291 w292] -> w287
              tunnel: w284 -> [w290 w292]
              tunnel: w283 -> [w289 _]
              tunnel: w280 -> [w288 _]
              frame True {
                n91 = invoke class="VI" method="FP.Open"(reference=w289, error in=w290, "State"=w288) -> (error out=w291:errorcluster)  [unwired: 2 in, 4 out]
              }
              frame False {
              }
            }
          }
          frame "Minimize", "Minimized" {
            w293 = T1."Minimized" ("State")
            n92 = property class="VI"(reference=w299, error in=w298) -> (reference out=w296:refnum<vi>, error out=w297:errorcluster, "FP.State"=w295:T1)
            n93 = Not Equal?(x=w295, y=w293) -> (x != y?=w294:bool)
            n94 = case shown="True" w294 {
              tunnel: [w304 w305] -> w300
              tunnel: w297 -> [w303 w305]
              tunnel: w296 -> [w302 _]
              tunnel: w293 -> [w301 _]
              frame True {
                n95 = invoke class="VI" method="FP.Open"(reference=w302, error in=w303, "State"=w301) -> (error out=w304:errorcluster)  [unwired: 2 in, 4 out]
              }
              frame False {
              }
            }
          }
          frame "Maximize", "Maximized" {
            w306 = T1."Maximized" ("State")
            n96 = property class="VI"(reference=w312, error in=w311) -> (reference out=w309:refnum<vi>, error out=w310:errorcluster, "FP.State"=w308:T1)
            n97 = Not Equal?(x=w308, y=w306) -> (x != y?=w307:bool)
            n98 = case shown="True" w307 {
              tunnel: [w317 w318] -> w313
              tunnel: w310 -> [w316 w318]
              tunnel: w309 -> [w315 _]
              tunnel: w306 -> [w314 _]
              frame True {
                n99 = invoke class="VI" method="FP.Open"(reference=w315, error in=w316, "State"=w314) -> (error out=w317:errorcluster)  [unwired: 2 in, 4 out]
              }
              frame False {
              }
            }
          }
        }
        n100 = call <vilib>:"Add State(s) to Queue__JKI_lib_State_Machine.vi"("State(s) in (\"\")"=w253) -> ("States Out"=w252:string)  [unwired: 14 in]
      }
      frame "---------- Macro ----------" {
        # "Do not put any code in this frame.\n(It is a separator no-op. You can make a copy of this frame to create a new Macro frame)"
        n101 = call <vilib>:"Add State(s) to Queue__JKI_lib_State_Machine.vi"("State(s) in (\"\")"=w323) -> ("States Out"=w322:string)  [unwired: 14 in]
      }
      frame "Macro: Initialize" {
        w325 = "Data: Initialize\nInitialize Core Data\nEvents: Register\nUI: Initialize\nUI: Front Panel State >> Open"  # Data: Initialize Initialize Core Data Events: Register UI: Initialize UI: Front Panel State >> Open
        # "Initialization Macro\n(This is called once, when the VI starts)"
        n102 = call <vilib>:"Add State(s) to Queue__JKI_lib_State_Machine.vi"("State(s) in Front (\"\")"=w325, "State(s) in (\"\")"=w329) -> ("States Out"=w328:string)  [unwired: 13 in]
      }
      frame "Macro: Exit" {
        # "Exit Macro\n(This is called once, when the VI exits)"
        n103 = Unbundle By Name(w337) -> ("Core.Close Panel on Exit?"=w336:bool)
        n104 = Select(t="UI: Front Panel State >> Close", s=w336, f="") -> (s? t:f=w333:string)
        n105 = call <vilib>:"Add State(s) to Queue__JKI_lib_State_Machine.vi"("State(s) in (\"\")"=w333, "State(s) at Back (\"\")"="Data: Cleanup\nEvents: Unregister\nExit") -> ("States Out"=w331:string)  [unwired: 13 in]
        n106 = call <vilib>:"Add State(s) to Queue__JKI_lib_State_Machine.vi"("State(s) in Front (\"\")"=w331, "State(s) in (\"\")"=w340) -> ("States Out"=w339:string)  [unwired: 13 in]
      }
      frame "---------- API ----------" {
        # "Do not put any code in this frame.\n(It is a separator no-op. This category is recommended to use for external API)"
      }
      frame "API: API1" {
        # "If you need to tell who triggered this state , use this string. If it's this case itself, this string is \"\"."
        # "Deal with the parameter if any"
        # "Connect this to return the response of your API"
        # "Copy/Rename this case for your own API"
      }
      frame "API: API2" {
        # "unpack HexStr  to Variant\nif complex parameter is needed."
        # "Copy/Rename this case for your own API"
        n107 = call "CSM - Convert HexStr to Data.vi"("HEX String"=w351) -> ()  [unwired: 7 in, 2 out]
        n108 = disable-structure shown="Disabled" {
          disable-tunnel: [w356 "API2 Response"] -> w350
          frame Disabled {
            # "pack variant to hexstr \nif complex response is needed."
            # "complex Response"
            n109 = call "CSM - Convert Data to HexStr.vi"() -> ("HEX String (0-9,A-F)"=w356:string)  [unwired: 9 in]
          }
          frame Enabled {
          }
        }
      }
      frame "---------- DoSth ----------" {
        # "Template Separator\n(You can make a copy of, or modify, this frame)"
        n110 = call <vilib>:"Add State(s) to Queue__JKI_lib_State_Machine.vi"("State(s) in (\"\")"=w362) -> ("States Out"=w361:string)  [unwired: 14 in]
      }
      frame "DoSth: DoA" {
        # "Your code here.\n(You can make a copy of, or modify, this frame)"
        n111 = call <vilib>:"Add State(s) to Queue__JKI_lib_State_Machine.vi"("State(s) in (\"\")"=w368) -> ("States Out"=w367:string)  [unwired: 14 in]
      }
      frame "Update Status Changed" {
        n112 = Format Into String(w371, w370) -> (resulting string=w369:string)  [unwired: 3 in, 1 out]
        n113 = call "String History Cacher.vi"("Include Timestamp? (T)"=TRUE ("Include Timestamp(F)"), "String"=w369) -> ("String Cache"=→"State History 2":string)  [unwired: 9 in]
      }
      frame "DoSth: DoB" {
        # "Your code here.\n(You can make a copy of, or modify, this frame)"
        n114 = call <vilib>:"Add State(s) to Queue__JKI_lib_State_Machine.vi"("State(s) in (\"\")"=w383) -> ("States Out"=w382:string)  [unwired: 14 in]
      }
      frame "Handler: Error Occurred" {
        n115 = Unbundle(w389) -> ("‘State"=w384:string)  [unwired: 2 out]
        n116 = call "CSM - Convert HexStr to Data.vi"("HEX String"=w395) -> ("Variant"=w394:variant)  [unwired: 7 in, 1 out]
        n117 = Variant To Data(type=errorcluster {"status"=FALSE, "code"=0, "source"=""} ("error in (no error)"), Variant=w394) -> (data=w392:errorcluster)  [unwired: 1 in, 1 out]
        n118 = Unbundle By Name(w392) -> ("source"=w391:string)
        n119 = Concatenate Strings("From:" ("string"), w390) -> (w388:string)
        n120 = Concatenate Strings("Because:" ("string"), w384) -> (w387:string)
        n121 = Two Button Dialog(message=w391, 1:w387, 2:w388) -> ()  [unwired: 1 out]
      }
    }
  }
